vi "Func-엑셀 데이터를 그래프로 출력.vi"() -> ()   [LabVIEW 2015] (continued)
-40\t-40\t-29.208\n-40\t-40\t-29.211\n-40\t-40\t-29.21\n-40\t-40\t-29.212\n-40\t-40\t-29.211\n-40\t-40\t-29.214\n-40\t-40\t-29.217\n-40\t-40\t-29.218\n-40\t-40\t-29.22\n-40\t-40\t-29.22\n-40\t-40\t-29.222\n-40\t-40\t-29.217\n-40\t-40\t-29.217\n-40\t-40\t-29.217\n-40\t-40\t-29.217\n-40\t-40\t-29.22\n-40\t-40\t-29.22\n-40\t-40\t-29.224\n-40\t-40\t-29.225\n-40\t-40\t-29.228\n-40\t-40\t-29.228\n-40\t-40\t-29.231\n-40\t-40\t-29.23\n-40\t-40\t-29.23\n-40\t-40\t-29.23\n-40\t-40\t-29.229\n-40\t-40\t-29.227\n-40\t-40\t-29.223\n-40\t-40\t-29.227\n-40\t-40\t-29.229\n-40\t-40\t-29.234\n-40\t-40\t-29.24\n-40\t-40\t-29.245\n-40\t-40\t-29.248\n-40\t-40\t-29.245\n-40\t-40\t-29.248\n-40\t-40\t-29.248\n-40\t-40\t-29.243\n-40\t-40\t-29.245\n-40\t-40\t-29.247\n-40\t-40\t-29.249\n-40\t-40\t-29.252\n-40\t-40\t-29.254\n-40\t-40\t-29.257\n-40\t-40\t-29.26\n-40\t-40\t-29.255\n-40\t-40\t-29.259\n-40\t-40\t-29.258\n-40\t-40\t-29.257\n-40\t-40\t-29.26\n-40\t-40\t-29.26\n-40\t-40\t-29.266\n-40\t-40\t-29.267\n-40\t-40\t-29.27\n-40\t-40\t-29.265\n-40\t-40\t-29.264\n-40\t-40\t-29.263\n-40\t-40\t-29.263\n-40\t-40\t-29.26\n-40\t-40\t-29.259\n-40\t-40\t-29.264\n-40\t-40\t-29.267\n-40\t-40\t-29.272\n-40\t-40\t-29.27\n-40\t-40\t-29.274\n-40\t-40\t-29.274\n-40\t-40\t-29.273\n-40\t-40\t-29.273\n-40\t-40\t-29.273\n-40\t-40\t-29.277\n-40\t-40\t-29.279\n-40\t-40\t-29.28\n-40\t-40\t-29.282\n-40\t-40\t-29.282\n-40\t-40\t-29.282\n-40\t-40\t-29.286\n-40\t-40\t-29.286\n-40\t-40\t-29.288\n-40\t-40\t-29.292\n-40\t-40\t-29.295\n-40\t-40\t-29.294\n-40\t-40\t-29.292\n-40\t-40\t-29.292\n-40\t-40\t-29.293\n-40\t-40\t-29.291\n-40\t-40\t-29.29\n-40\t-40\t-29.291\n-40\t-40\t-29.292\n-40\t-40\t-29.295\n-40\t-40\t-29.295\n-40\t-40\t-29.297\n-40\t-40\t-29.298\n-40\t-40\t-29.3\n-40\t-40\t-29.301\n-40\t-40\t-29.3\n-40\t-40\t-29.303\n-40\t-40\t-29.305\n-40\t-40\t-29.307\n-40\t-40\t-29.307\n-40\t-40\t-29.307\n-40\t-40\t-29.312\n-40\t-40\t-29.311\n-40\t-40\t-29.311\n-40\t-40\t-29.311\n-40\t-40\t-29.314\n-40\t-40\t-29.316\n-40\t-40\t-29.312\n-40\t-40\t-29.314\n-40\t-40\t-29.315\n-40\t-40\t-29.315\n-40\t-40\t-29.315\n-40\t-40\t-29.314\n-40\t-40\t-29.318\n-40\t-40\t-29.318\n-40\t-40\t-29.32\n-40\t-40\t-29.322\n-40\t-40\t-29.323\n-40\t-40\t-29.324\n-40\t-40\t-29.326\n-40\t-40\t-29.329\n-40\t-40\t-29.329\n-40\t-40\t-29.328\n-40\t-40\t-29.33\n-40\t-40\t-29.336\n-40\t-40\t-29.336\n-40\t-40\t-29.336\n-40\t-40\t-29.336\n-40\t-40\t-29.339\n-40\t-40\t-29.336\n-40\t-40\t-29.333\n-40\t-40\t-29.334\n-40\t-40\t-29.333\n-40\t-40\t-29.332\n-40\t-40\t-29.331\n-40\t-40\t-29.33\n-40\t-40\t-29.329\n-40\t-40\t-29.328\n-40\t-40\t-29.33\n-40\t-40\t-29.333\n-40\t-40\t-29.337\n-40\t-40\t-29.343\n-40\t-40\t-29.348\n-40\t-40\t-29.351\n-40\t-40\t-29.351\n-40\t-40\t-29.35\n-40\t-40\t-29.35\n-40\t-40\t-29.351\n-40\t-40\t-29.35\n-40\t-40\t-29.35\n-40\t-40\t-29.351\n-40\t-40\t-29.352\n-40\t-40\t-29.35\n-40\t-40\t-29.35\n-40\t-40\t-29.352\n-40\t-40\t-29.353\n-40\t-40\t-29.352\n-40\t-40\t-29.355\n-40\t-40\t-29.359\n-40\t-40\t-29.36\n-40\t-40\t-29.357\n-40\t-40\t-29.361\n-40\t-40\t-29.364\n-40\t-40\t-29.362\n-40\t-40\t-29.366\n-40\t-40\t-29.363\n-40\t-40\t-29.367\n-40\t-40\t-29.37\n-40\t-40\t-29.372\n-40\t-40\t-29.376\n-40\t-40\t-29.375\n-40\t-40\t-29.376\n-40\t-40\t-29.375\n-40\t-40\t-29.373\n-40\t-40\t-29.37\n-40\t-40\t-29.368\n-40\t-40\t-29.368\n-40\t-40\t-29.371\n-40\t-40\t-29.376\n-40\t-40\t-29.377\n-40\t-40\t-29.377\n-40\t-40\t-29.377\n-40\t-40\t-29.378\n-40\t-40\t-29.382\n-40\t-40\t-29.38\n-40\t-40\t-29.385\n-40\t-40\t-29.389\n-40\t-40\t-29.394\n-40\t-40\t-29.396\n-40\t-40\t-29.391\n-40\t-40\t-29.392\n-40\t-40\t-29.389\n-40\t-40\t-29.39\n-40\t-40\t-29.388\n-40\t-40\t-29.388\n-40\t-40\t-29.389\n-40\t-40\t-29.39\n-40\t-40\t-29.391\n-40\t-40\t-29.393\n-40\t-40\t-29.396\n-40\t-40\t-29.396\n-40\t-40\t-29.397\n-40\t-40\t-29.4\n-40\t-40\t-29.4\n-40\t-40\t-29.4\n-40\t-40\t-29.403\n-40\t-40\t-29.406\n-40\t-40\t-29.409\n-40\t-40\t-29.41\n-40\t-40\t-29.412\n-40\t-40\t-29.411\n-40\t-40\t-29.411\n-40\t-40\t-29.413\n-40\t-40\t-29.414\n-40\t-40\t-29.412\n-40\t-40\t-29.414\n-40\t-40\t-29.415\n-40\t-40\t-29.415\n-40\t-40\t-29.412\n-40\t-40\t-29.41\n-40\t-40\t-29.413\n-40\t-40\t-29.414\n-40\t-40\t-29.414\n-40\t-40\t-29.413\n-40\t-40\t-29.414\n-40\t-40\t-29.417\n-40\t-40\t-29.418\n-40\t-40\t-29.419\n-40\t-40\t-29.423\n-40\t-40\t-29.427\n-40\t-40\t-29.428\n-40\t-40\t-29.429\n-40\t-40\t-29.429\n-40\t-40\t-29.429\n-40\t-40\t-29.426\n-40\t-40\t-29.425\n-40\t-40\t-29.427\n-40\t-40\t-29.426\n-40\t-40\t-29.428\n-40\t-40\t-29.427\n-40\t-40\t-29.43\n-40\t-40\t-29.43\n-40\t-40\t-29.43\n-40\t-40\t-29.43\n-40\t-40\t-29.43\n-40\t-40\t-29.432\n-40\t-40\t-29.431\n-40\t-40\t-29.434\n-40\t-40\t-29.432\n-40\t-40\t-29.432\n-40\t-40\t-29.432\n-40\t-40\t-29.433\n-40\t-40\t-29.435\n-40\t-40\t-29.439\n-40\t-40\t-29.437\n-40\t-40\t-29.44\n-40\t-40\t-29.442\n-40\t-40\t-29.442\n-40\t-40\t-29.441\n-40\t-40\t-29.44\n-40\t-40\t-29.445\n-40\t-40\t-29.446\n-40\t-40\t-29.448\n-40\t-40\t-29.446\n-40\t-40\t-29.445\n-40\t-40\t-29.445\n-40\t-40\t-29.447\n-40\t-40\t-29.447\n-40\t-40\t-29.445\n-40\t-40\t-29.447\n-40\t-40\t-29.448\n-40\t-40\t-29.45\n-40\t-40\t-29.445\n-40\t-40\t-29.448\n-40\t-40\t-29.451\n-40\t-40\t-29.452\n-40\t-40\t-29.459\n-40\t-40\t-29.458\n-40\t-40\t-29.462\n-40\t-40\t-29.462\n-40\t-40\t-29.459\n-40\t-40\t-29.462\n-40\t-40\t-29.458\n-40\t-40\t-29.463\n-40\t-40\t-29.459\n-40\t-40\t-29.459\n-40\t-40\t-29.462\n-40\t-40\t-29.462\n-40\t-40\t-29.465\n-40\t-40\t-29.461\n-40\t-40\t-29.464\n-40\t-40\t-29.467\n-40\t-40\t-29.47\n-40\t-40\t-29.472\n-40\t-40\t-29.472\n-40\t-40\t-29.475\n-40\t-40\t-29.478\n-40\t-40\t-29.477\n-40\t-40\t-29.475\n-40\t-40\t-29.475\n-40\t-40\t-29.476\n-40\t-40\t-29.48\n-40\t-40\t-29.482\n-40\t-40\t-29.484\n-40\t-40\t-29.483\n-40\t-40\t-29.485\n-40\t-40\t-29.483\n-40\t-40\t-29.482\n-40\t-40\t-29.479\n-40\t-40\t-29.48\n-40\t-40\t-29.48\n-40\t-40\t-29.478\n-40\t-40\t-29.48\n-40\t-40\t-29.482\n-40\t-40\t-29.486\n-40\t-40\t-29.485\n-40\t-40\t-29.484\n-40\t-40\t-29.487\n-40\t-40\t-29.489\n-40\t-40\t-29.487\n-40\t-40\t-29.484\n-40\t-40\t-29.487\n-40\t-40\t-29.492\n-40\t-40\t-29.492\n-40\t-40\t-29.488\n-40\t-40\t-29.49\n-40\t-40\t-29.489\n-40\t-40\t-29.49\n-40\t-40\t-29.492\n-40\t-40\t-29.495\n-40\t-40\t-29.497\n-40\t-40\t-29.499\n-40\t-40\t-29.502\n-40\t-40\t-29.498\n-40\t-40\t-29.495\n-40\t-40\t-29.492\n-40\t-40\t-29.496\n-40\t-40\t-29.499\n-40\t-40\t-29.501\n-40\t-40\t-29.504\n-40\t-40\t-29.507\n-40\t-40\t-29.508\n-40\t-40\t-29.509\n-40\t-40\t-29.507\n-40\t-40\t-29.508\n-40\t-40\t-29.509\n-40\t-40\t-29.51\n-40\t-40\t-29.511\n-40\t-40\t-29.51\n-40\t-40\t-29.508\n-40\t-40\t-29.507\n-40\t-40\t-29.508\n-40\t-40\t-29.508\n-40\t-40\t-29.51\n-40\t-40\t-29.51\n-40\t-40\t-29.511\n-40\t-40\t-29.51\n-40\t-40\t-29.512\n-40\t-40\t-29.514\n-40\t-40\t-29.515\n-40\t-40\t-29.516\n-40\t-40\t-29.523\n-40\t-40\t-29.524\n-40\t-40\t-29.523\n-40\t-40\t-29.52\n-40\t-40\t-29.521\n-40\t-40\t-29.519\n-40\t-40\t-29.517\n-40\t-40\t-29.516\n-40\t-40\t-29.517\n-40\t-40\t-29.521\n-40\t-40\t-29.52\n-40\t-40\t-29.524\n-40\t-40\t-29.524\n-40\t-40\t-29.53\n-40\t-40\t-29.53\n-40\t-40\t-29.529\n-40\t-40\t-29.531\n-40\t-40\t-29.533\n-40\t-40\t-29.532\n-40\t-40\t-29.532\n-40\t-40\t-29.53\n-40\t-40\t-29.533\n-40\t-40\t-29.533\n-40\t-40\t-29.531\n-40\t-40\t-29.531\n-40\t-40\t-29.532\n-40\t-40\t-29.534\n-40\t-40\t-29.532\n-40\t-40\t-29.534\n-40\t-40\t-29.538\n-40\t-40\t-29.544\n-40\t-40\t-29.542\n-40\t-40\t-29.543\n-40\t-40\t-29.547\n-40\t-40\t-29.543\n-40\t-40\t-29.541\n-40\t-40\t-29.538\n-40\t-40\t-29.542\n-40\t-40\t-29.543\n-40\t-40\t-29.543\n-40\t-40\t-29.547\n-40\t-40\t-29.546\n-40\t-40\t-29.548\n-40\t-40\t-29.545\n-40\t-40\t-29.544\n-40\t-40\t-29.543\n-40\t-40\t-29.546\n-40\t-40\t-29.549\n-40\t-40\t-29.548\n-40\t-40\t-29.553\n-40\t-40\t-29.552\n-40\t-40\t-29.554\n-40\t-40\t-29.554\n-40\t-40\t-29.554\n-40\t-40\t-29.555\n-40\t-40\t-29.553\n-40\t-40\t-29.553\n-40\t-40\t-29.55\n-40\t-40\t-29.55\n-40\t-40\t-29.554\n-40\t-40\t-29.553\n-40\t-40\t-29.552\n-40\t-40\t-29.553\n-40\t-40\t-29.556\n-40\t-40\t-29.557\n-40\t-40\t-29.555\n-40\t-40\t-29.557\n-40\t-40\t-29.558\n-40\t-40\t-29.562\n-40\t-40\t-29.559\n-40\t-40\t-29.56\n-40\t-40\t-29.56\n-40\t-40\t-29.559\n-40\t-40\t-29.56\n-40\t-40\t-29.56\n-40\t-40\t-29.562\n-40\t-40\t-29.562\n-40\t-40\t-29.564\n-40\t-40\t-29.562\n-40\t-40\t-29.561\n-40\t-40\t-29.563\n-40\t-40\t-29.564\n-40\t-40\t-29.564\n-40\t-40\t-29.564\n-40\t-40\t-29.571\n-40\t-40\t-29.573\n-40\t-40\t-29.575\n-40\t-40\t-29.578\n-40\t-40\t-29.579\n-40\t-40\t-29.578\n-40\t-40\t-29.573\n-40\t-40\t-29.572\n-40\t-40\t-29.574\n-40\t-40\t-29.571\n-40\t-40\t-29.572\n-40\t-40\t-29.574\n-40\t-40\t-29.58\n-40\t-40\t-29.582\n-40\t-40\t-29.58\n-40\t-40\t-29.582\n-40\t-40\t-29.582\n-40\t-40\t-29.582\n-40\t-40\t-29.585\n-40\t-40\t-29.584\n-40\t-40\t-29.585\n-40\t-40\t-29.584\n-40\t-40\t-29.587\n-40\t-40\t-29.587\n-40\t-40\t-29.587\n-40\t-40\t-29.587\n-40\t-40\t-29.589\n-40\t-40\t-29.59\n-40\t-40\t-29.585\n-40\t-40\t-29.586\n-40\t-40\t-29.582\n-40\t-40\t-29.582\n-40\t-40\t-29.583\n-40\t-40\t-29.584\n-40\t-40\t-29.587\n-40\t-40\t-29.586\n-40\t-40\t-29.59\n-40\t-40\t-29.594\n-40\t-40\t-29.595\n-40\t-40\t-29.595\n-40\t-40\t-29.594\n-40\t-40\t-29.596\n-39.917\t-39.94\t-29.897\n-39.833\t-39.88\t-29.901\n-39.75\t-40.02\t-29.899\n-39.667\t-40.02\t-29.901\n-39.583\t-40.03\t-29.901\n-39.5\t-40.05\t-29.911\n-39.417\t-40.06\t-29.912\n-39.333\t-40.06\t-29.916\n-39.25\t-40.05\t-29.915\n-39.167\t-40.04\t-29.92\n-39.083\t-40.02\t-29.922\n-39\t-40\t-29.918\n-38.917\t-39.97\t-29.922\n-38.833\t-39.95\t-29.926\n-38.75\t-39.92\t-29.923\n-38.667\t-39.87\t-29.932\n-38.583\t-39.82\t-29.933\n-38.5\t-39.76\t-29.929\n-38.417\t-39.71\t-29.932\n-38.333\t-39.65\t-29.937\n-38.25\t-39.58\t-29.938\n-38.167\t-39.5\t-29.939\n-38.083\t-39.42\t-29.936\n-38\t-39.34\t-29.938\n-37.917\t-39.25\t-29.937\n-37.833\t-39.16\t-29.935\n-37.75\t-39.08\t-29.936\n-37.667\t-39\t-29.942\n-37.583\t-38.91\t-29.936\n-37.5\t-38.83\t-29.939\n-37.417\t-38.75\t-29.934\n-37.333\t-38.67\t-29.936\n-37.25\t-38.58\t-29.932\n-37.167\t-38.49\t-29.925\n-37.083\t-38.4\t-29.927\n-37\t-38.32\t-29.923\n-36.917\t-38.23\t-29.916\n-36.833\t-38.15\t-29.914\n-36.75\t-38.06\t-29.913\n-36.667\t-37.99\t-29.901\n-36.583\t-37.9\t-29.89\n-36.5\t-37.81\t-29.888\n-36.417\t-37.72\t-29.886\n-36.333\t-37.63\t-29.879\n-36.25\t-37.57\t-29.864\n-36.167\t-37.49\t-29.853\n-36.083\t-37.4\t-29.843\n-36\t-37.32\t-29.834\n-35.917\t-37.24\t-29.821\n-35.833\t-37.16\t-29.802\n-35.75\t-37.08\t-29.796\n-35.667\t-37\t-29.787\n-35.583\t-36.91\t-29.767\n-35.5\t-36.83\t-29.75\n-35.417\t-36.75\t-29.733\n-35.333\t-36.67\t-29.718\n-35.25\t-36.58\t-29.7\n-35.167\t-36.5\t-29.682\n-35.083\t-36.42\t-29.662\n-35\t-36.35\t-29.645\n-34.917\t-36.28\t-29.631\n-34.833\t-36.2\t-29.607\n-34.75\t-36.12\t-29.589\n-34.667\t-36.05\t-29.573\n-34.583\t-35.97\t-29.558\n-34.5\t-35.89\t-29.529\n-34.417\t-35.8\t-29.509\n-34.333\t-35.72\t-29.497\n-34.25\t-35.64\t-29.47\n-34.167\t-35.56\t-29.445\n-34.083\t-35.48\t-29.426\n-34\t-35.39\t-29.403\n-33.917\t-35.31\t-29.383\n-33.833\t-35.23\t-29.355\n-33.75\t-35.15\t-29.338\n-33.667\t-35.08\t-29.316\n-33.583\t-35\t-29.293\n-33.5\t-34.93\t-29.263\n-33.417\t-34.86\t-29.241\n-33.333\t-34.78\t-29.219\n-33.25\t-34.71\t-29.195\n-33.167\t-34.63\t-29.173\n-33.083\t-34.55\t-29.143\n-33\t-34.47\t-29.117\n-32.917\t-34.4\t-29.084\n-32.833\t-34.32\t-29.065\n-32.75\t-34.24\t-29.028\n-32.667\t-34.16\t-29.002\n-32.583\t-34.08\t-28.978\n-32.5\t-33.99\t-28.935\n-32.417\t-33.9\t-28.909\n-32.333\t-33.83\t-28.877\n-32.25\t-33.75\t-28.841\n-32.167\t-33.67\t-28.806\n-32.083\t-33.59\t-28.772\n-32\t-33.51\t-28.735\n-31.917\t-33.44\t-28.705\n-31.833\t-33.36\t-28.661\n-31.75\t-33.27\t-28.631\n-31.667\t-33.19\t-28.588\n-31.583\t-33.11\t-28.554\n-31.5\t-33.03\t-28.509\n-31.417\t-32.96\t-28.47\n-31.333\t-32.89\t-28.427\n-31.25\t-32.81\t-28.395\n-31.167\t-32.73\t-28.353\n-31.083\t-32.65\t-28.305\n-31\t-32.56\t-28.263\n-30.917\t-32.49\t-28.227\n-30.833\t-32.42\t-28.176\n-30.75\t-32.32\t-28.142\n-30.667\t-32.25\t-28.088\n-30.583\t-32.17\t-28.05\n-30.5\t-32.09\t-28.001\n-30.417\t-32\t-27.954\n-30.333\t-31.93\t-27.908\n-30.25\t-31.84\t-27.861\n-30.167\t-31.76\t-27.817\n-30.083\t-31.68\t-27.773\n-30\t-31.6\t-27.72\n-29.917\t-31.52\t-27.671\n-29.833\t-31.44\t-27.621\n-29.75\t-31.35\t-27.573\n-29.667\t-31.28\t-27.521\n-29.583\t-31.2\t-27.473\n-29.5\t-31.12\t-27.426\n-29.417\t-31.04\t-27.371\n-29.333\t-30.96\t-27.332\n-29.25\t-30.89\t-27.273\n-29.167\t-30.81\t-27.224\n-29.083\t-30.73\t-27.171\n-29\t-30.64\t-27.115\n-28.917\t-30.57\t-27.066\n-28.833\t-30.49\t-27.007\n-28.75\t-30.4\t-26.954\n-28.667\t-30.32\t-26.894\n-28.583\t-30.24\t-26.844\n-28.5\t-30.16\t-26.802\n-28.417\t-30.09\t-26.743\n-28.333\t-30.02\t-26.686\n-28.25\t-29.94\t-26.632\n-28.167\t-29.87\t-26.564\n-28.083\t-29.79\t-26.515\n-28\t-29.72\t-26.456\n-27.917\t-29.64\t-26.398\n-27.833\t-29.57\t-26.341\n-27.75\t-29.48\t-26.289\n-27.667\t-29.4\t-26.23\n-27.583\t-29.31\t-26.174\n-27.5\t-29.23\t-26.114\n-27.417\t-29.14\t-26.062\n-27.333\t-29.07\t-25.995\n-27.25\t-28.97\t-25.941\n-27.167\t-28.89\t-25.886\n-27.083\t-28.81\t-25.823\n-27\t-28.74\t-25.761\n-26.917\t-28.65\t-25.698\n-26.833\t-28.57\t-25.638\n-26.75\t-28.5\t-25.585\n-26.667\t-28.43\t-25.525\n-26.583\t-28.35\t-25.456\n-26.5\t-28.28\t-25.401\n-26.417\t-28.2\t-25.339\n-26.333\t-28.12\t-25.275\n-26.25\t-28.04\t-25.22\n-26.167\t-27.97\t-25.155\n-26.083\t-27.89\t-25.092\n-26\t-27.81\t-25.03\n-25.917\t-27.74\t-24.968\n-25.833\t-27.65\t-24.902\n-25.75\t-27.57\t-24.847\n-25.667\t-27.49\t-24.787\n-25.583\t-27.42\t-24.723\n-25.5\t-27.34\t-24.656\n-25.417\t-27.26\t-24.595\n-25.333\t-27.17\t-24.528\n-25.25\t-27.09\t-24.46\n-25.167\t-27.01\t-24.404\n-25.083\t-26.92\t-24.334\n-25\t-26.85\t-24.267\n-24.917\t-26.77\t-24.21\n-24.833\t-26.69\t-24.145\n-24.75\t-26.62\t-24.092\n-24.667\t-26.53\t-24.016\n-24.583\t-26.46\t-23.95\n-24.5\t-26.38\t-23.886\n-24.417\t-26.29\t-23.822\n-24.333\t-26.21\t-23.753\n-24.25\t-26.13\t-23.683\n-24.167\t-26.05\t-23.627\n-24.083\t-25.97\t-23.556\n-24\t-25.89\t-23.49\n-23.917\t-25.81\t-23.43\n-23.833\t-25.74\t-23.357\n-23.75\t-25.66\t-23.295\n-23.667\t-25.58\t-23.228\n-23.583\t-25.5\t-23.163\n-23.5\t-25.42\t-23.094\n-23.417\t-25.34\t-23.026\n-23.333\t-25.26\t-22.961\n-23.25\t-25.19\t-22.894\n-23.167\t-25.11\t-22.832\n-23.083\t-25.03\t-22.76\n-23\t-24.94\t-22.696\n-22.917\t-24.86\t-22.624\n-22.833\t-24.78\t-22.566\n-22.75\t-24.7\t-22.488\n-22.667\t-24.62\t-22.416\n-22.583\t-24.54\t-22.358\n-22.5\t-24.47\t-22.288\n-22.417\t-24.38\t-22.215\n-22.333\t-24.29\t-22.145\n-22.25\t-24.21\t-22.077\n-22.167\t-24.14\t-22.007\n-22.083\t-24.06\t-21.939\n-22\t-23.98\t-21.874\n-21.917\t-23.9\t-21.804\n-21.833\t-23.82\t-21.738\n-21.75\t-23.74\t-21.668\n-21.667\t-23.66\t-21.597\n-21.583\t-23.58\t-21.525\n-21.5\t-23.51\t-21.461\n-21.417\t-23.42\t-21.39\n-21.333\t-23.35\t-21.324\n-21.25\t-23.27\t-21.255\n-21.167\t-23.19\t-21.176\n-21.083\t-23.11\t-21.107\n-21\t-23.03\t-21.045\n-20.917\t-22.95\t-20.975\n-20.833\t-22.87\t-20.905\n-20.75\t-22.8\t-20.835\n-20.667\t-22.72\t-20.761\n-20.583\t-22.63\t-20.693\n-20.5\t-22.55\t-20.626\n-20.417\t-22.47\t-20.55\n-20.333\t-22.39\t-20.475\n-20.25\t-22.32\t-20.407\n-20.167\t-22.24\t-20.335\n-20.083\t-22.15\t-20.262\n-20\t-22.07\t-20.192\n-19.917\t-21.99\t-20.133\n-19.833\t-21.91\t-20.058\n-19.75\t-21.84\t-19.984\n-19.667\t-21.75\t-19.909\n-19.583\t-21.68\t-19.836\n-19.5\t-21.59\t-19.77\n-19.417\t-21.51\t-19.694\n-19.333\t-21.44\t-19.628\n-19.25\t-21.37\t-19.559\n-19.167\t-21.29\t-19.483\n-19.083\t-21.22\t-19.411\n-19\t-21.14\t-19.341\n-18.917\t-21.07\t-19.266\n-18.833\t-20.99\t-19.192\n-18.75\t-20.91\t-19.12\n-18.667\t-20.83\t-19.047\n-18.583\t-20.76\t-18.987\n-18.5\t-20.69\t-18.905\n-18.417\t-20.61\t-18.83\n-18.3\t-20.55\t-18.77\n-18.3\t-20.54\t-18.767\n-18.3\t-20.53\t-18.757\n-18.3\t-20.52\t-18.748\n-18.3\t-20.52\t-18.742\n-18.3\t-20.51\t-18.737\n-18.3\t-20.5\t-18.731\n-18.3\t-20.49\t-18.721\n-18.3\t-20.48\t-18.712\n-18.3\t-20.47\t-18.705\n-18.3\t-20.46\t-18.698\n-18.3\t-20.45\t-18.692\n-18.3\t-20.45\t-18.683\n-18.3\t-20.44\t-18.675\n-18.3\t-20.43\t-18.672\n-18.3\t-20.42\t-18.664\n-18.3\t-20.41\t-18.657\n-18.3\t-20.4\t-18.651\n-18.3\t-20.4\t-18.641\n-18.3\t-20.39\t-18.639\n-18.3\t-20.38\t-18.629\n-18.3\t-20.38\t-18.624\n-18.3\t-20.37\t-18.62\n-18.3\t-20.36\t-18.613\n-18.3\t-20.35\t-18.604\n-18.3\t-20.34\t-18.598\n-18.3\t-20.33\t-18.587\n-18.3\t-20.33\t-18.58\n-18.3\t-20.32\t-18.573\n-18.3\t-20.32\t-18.565\n-18.3\t-20.31\t-18.558\n-18.3\t-20.3\t-18.55\n-18.3\t-20.29\t-18.542\n-18.3\t-20.28\t-18.531\n-18.3\t-20.27\t-18.522\n-18.3\t-20.26\t-18.514\n-18.3\t-20.25\t-18.508\n-18.3\t-20.25\t-18.502\n-18.3\t-20.25\t-18.497\n-18.3\t-20.24\t-18.493\n-18.3\t-20.23\t-18.484\n-18.3\t-20.22\t-18.472\n-18.3\t-20.21\t-18.466\n-18.3\t-20.2\t-18.457\n-18.3\t-20.19\t-18.447\n-18.3\t-20.19\t-18.44\n-18.3\t-20.18\t-18.438\n-18.3\t-20.17\t-18.431\n-18.3\t-20.17\t-18.429\n-18.3\t-20.17\t-18.425\n-18.3\t-20.16\t-18.418\n-18.3\t-20.15\t-18.413\n-18.3\t-20.14\t-18.405\n-18.3\t-20.13\t-18.394\n-18.3\t-20.12\t-18.385\n-18.3\t-20.12\t-18.376\n-18.3\t-20.11\t-18.362\n-18.3\t-20.1\t-18.355\n-18.3\t-20.09\t-18.349\n-18.3\t-20.09\t-18.344\n-18.3\t-20.09\t-18.335\n-18.3\t-20.08\t-18.332\n-18.3\t-20.07\t-18.327\n-18.3\t-20.06\t-18.324\n-18.3\t-20.05\t-18.316\n-18.3\t-20.04\t-18.309\n-18.3\t-20.03\t-18.303\n-18.3\t-20.02\t-18.293\n-18.3\t-20.01\t-18.284\n-18.3\t-20.01\t-18.274\n-18.3\t-20\t-18.27\n-18.3\t-19.99\t-18.259\n-18.3\t-19.99\t-18.252\n-18.3\t-19.98\t-18.243\n-18.3\t-19.97\t-18.238\n-18.3\t-19.96\t-18.231\n-18.3\t-19.96\t-18.222\n-18.3\t-19.95\t-18.214\n-18.3\t-19.94\t-18.206\n-18.3\t-19.93\t-18.199\n-18.3\t-19.93\t-18.191\n-18.3\t-19.93\t-18.187\n-18.3\t-19.92\t-18.179\n-18.3\t-19.91\t-18.17\n-18.3\t-19.91\t-18.166\n-18.3\t-19.9\t-18.155\n-18.3\t-19.89\t-18.148\n-18.3\t-19.88\t-18.142\n-18.3\t-19.88\t-18.137\n-18.3\t-19.87\t-18.132\n-18.3\t-19.86\t-18.127\n-18.3\t-19.85\t-18.12\n-18.3\t-19.85\t-18.116\n-18.3\t-19.85\t-18.105\n-18.3\t-19.85\t-18.095\n-18.3\t-19.84\t-18.087\n-18.3\t-19.83\t-18.081\n-18.3\t-19.82\t-18.071\n-18.3\t-19.81\t-18.063\n-18.3\t-19.8\t-18.059\n-18.3\t-19.8\t-18.051\n-18.3\t-19.79\t-18.045\n-18.3\t-19.79\t-18.04\n-18.3\t-19.78\t-18.03\n-18.3\t-19.78\t-18.023\n-18.3\t-19.77\t-18.015\n-18.3\t-19.76\t-18.004\n-18.3\t-19.76\t-17.996\n-18.3\t-19.75\t-17.985\n-18.3\t-19.74\t-17.977\n-18.3\t-19.74\t-17.971\n-18.3\t-19.73\t-17.964\n-18.3\t-19.72\t-17.957\n-18.3\t-19.72\t-17.954\n-18.3\t-19.71\t-17.949\n-18.3\t-19.7\t-17.943\n-18.3\t-19.69\t-17.939\n-18.3\t-19.69\t-17.934\n-18.3\t-19.69\t-17.924\n-18.3\t-19.68\t-17.913\n-18.3\t-19.67\t-17.907\n-18.3\t-19.66\t-17.896\n-18.3\t-19.65\t-17.889\n-18.3\t-19.64\t-17.88\n-18.3\t-19.63\t-17.872\n-18.3\t-19.62\t-17.869\n-18.3\t-19.62\t-17.859\n-18.3\t-19.61\t-17.85\n-18.3\t-19.61\t-17.844\n-18.3\t-19.6\t-17.84\n-18.3\t-19.59\t-17.835\n-18.3\t-19.58\t-17.827\n-18.3\t-19.57\t-17.818\n-18.3\t-19.57\t-17.814\n-18.3\t-19.56\t-17.808\n-18.3\t-19.55\t-17.803\n-18.3\t-19.54\t-17.794\n-18.3\t-19.53\t-17.788\n-18.3\t-19.53\t-17.784\n-18.3\t-19.52\t-17.778\n-18.3\t-19.52\t-17.768\n-18.3\t-19.51\t-17.756\n-18.3\t-19.5\t-17.745\n-18.3\t-19.49\t-17.741\n-18.3\t-19.49\t-17.731\n-18.3\t-19.48\t-17.722\n-18.3\t-19.47\t-17.716\n-18.3\t-19.46\t-17.711\n-18.3\t-19.46\t-17.707\n-18.3\t-19.46\t-17.696\n-18.3\t-19.45\t-17.686\n-18.3\t-19.44\t-17.68\n-18.3\t-19.43\t-17.674\n-18.3\t-19.43\t-17.664\n-18.3\t-19.42\t-17.656\n-18.3\t-19.41\t-17.652\n-18.3\t-19.4\t-17.645\n-18.3\t-19.4\t-17.636\n-18.3\t-19.39\t-17.632\n-18.3\t-19.39\t-17.621\n-18.3\t-19.38\t-17.613\n-18.3\t-19.37\t-17.602\n-18.3\t-19.37\t-17.593\n-18.3\t-19.36\t-17.591\n-18.3\t-19.36\t-17.58\n-18.3\t-19.35\t-17.573\n-18.3\t-19.34\t-17.57\n-18.3\t-19.33\t-17.563\n-18.3\t-19.32\t-17.554\n-18.3\t-19.32\t-17.545\n-18.3\t-19.31\t-17.539\n-18.3\t-19.31\t-17.531\n-18.3\t-19.3\t-17.523\n-18.3\t-19.3\t-17.521\n-18.3\t-19.29\t-17.509\n-18.3\t-19.28\t-17.503\n-18.3\t-19.28\t-17.5\n-18.3\t-19.27\t-17.491\n-18.3\t-19.27\t-17.487\n-18.3\t-19.26\t-17.477\n-18.3\t-19.26\t-17.471\n-18.3\t-19.25\t-17.464\n-18.3\t
